vi "Get Mandatory Objects List.vi"(8 "error in":errorcluster, 11 "EDS in":refnum<class "EDS.lvclass">) -> (0 "error out":errorcluster, 2 "Objects List":string[](array[string]), 3 "EDS out":refnum<class "EDS.lvclass">)   [LabVIEW 2024, in "EDS.lvlib" / "EDS.lvclass"]
uses:
  EDS.lvclass
  EDS.lvclass/EDS.ctl
  OD Section/Section.lvclass/Section.ctl
  Object Dictionary/Dictionary.lvclass
  OD Section/Section.lvclass
  Value/Value.lvclass
  Keyname/Key Name.lvclass
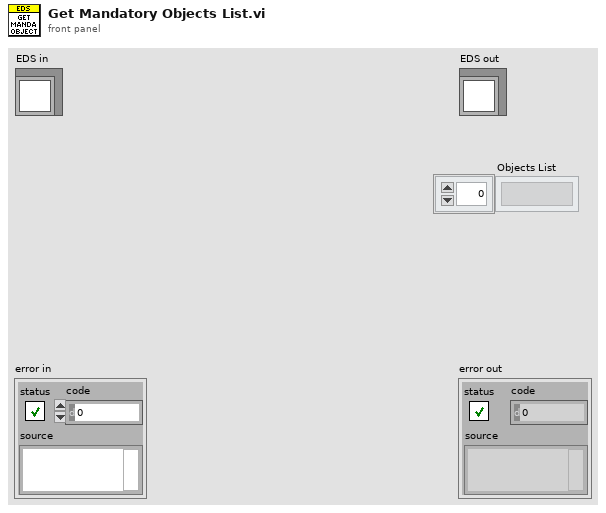
[diagram p1: front panel]
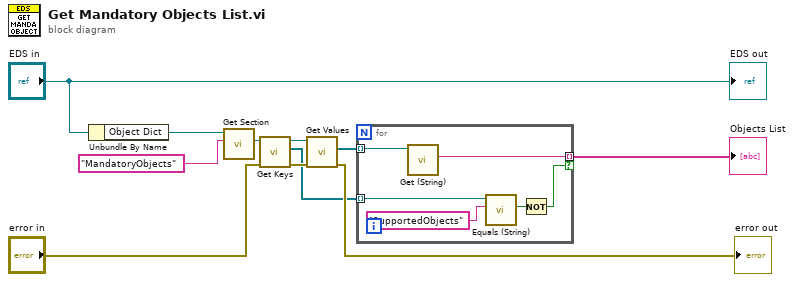
[diagram p0: block diagram]
diagram:
  n1 = Unbundle By Name("EDS in") -> ("Object Dict"=w10:refnum<class "Dictionary.lvclass">)
  n2 = call "Get Section.vi"("Section"="MandatoryObjects", "Dictionary in"=w10) -> ("Section out"=w3:refnum<class "Section.lvclass">)  [unwired: 7 in, 2 out]
  n3 = call "Get Keys.vi"("error in"="error in", "Object Entry in"=w3) -> ("error out"=w4:errorcluster, "Keys"=w1:refnum<class "Key Name.lvclass">[], "Object Entry out"=w2:refnum<class "Section.lvclass">)  [unwired: 7 in]
  n4 = call "Get Values.vi"("error in (no error)"=w4, "Section in"=w2) -> ("error out"=→"error out":errorcluster, "Values"=w6:refnum<class "Value.lvclass">[])  [unwired: 7 in, 1 out]
  n5 = for {
    tunnel: w6 -> [w17] mode=indexing
    tunnel: [w16] -> w5 mode=indexing if=w12
    tunnel: w1 -> [w15] mode=indexing
    n6 = call "Get (String).vi"("Value in"=w17) -> ("Value"=w16:string)  [unwired: 8 in, 2 out]
    n7 = call "Equals (String).vi"("Keyname"="SupportedObjects", "Keyname in"=w15) -> ("Equal?"=w13:bool)  [unwired: 8 in, 1 out]
    n8 = Not(x=w13) -> (.not. x?=w12:bool)
  }
  "Objects List" <- w5
  "EDS out" <- "EDS in"
